vi "Init Headers (raw string).vi"(5 "httpHeaders in":refnum<class "httpHeaders.lvclass">, 10 "headers":cluster{"header":string, "value":string}[](array[cluster])) -> (3 "httpHeaders out":refnum<class "httpHeaders.lvclass">)   [LabVIEW 2020]
uses:
  httpHeaders.lvclass
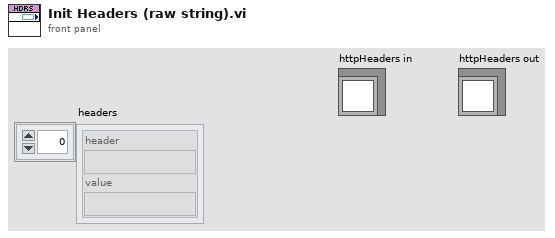
[diagram p1: front panel]
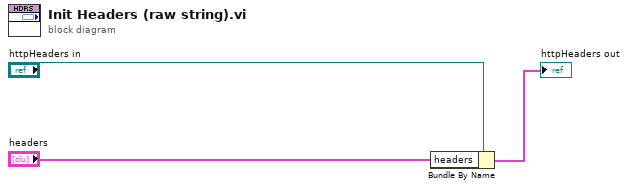
[diagram p0: block diagram]
diagram:
  n1 = Bundle By Name(cluster="httpHeaders in", "headers"="headers") -> (→"httpHeaders out":cluster{})
